vi "PI with FF_0.vi"(0 "Run PI?":bool, 1 "PIcluster":cluster{"SlewRate":dbl, "Kp":dbl, "Ki":dbl}, 2 "FFcluster":cluster{"FF_m":dbl, "FF_b":dbl}, 3 "LimitCluster":T1, 5 "SP":dbl, 7 "Error":dbl, 11 "RevCtrlZero":bool, 13 "Indirect FF":bool) -> (4 "PreSlew":dbl, 8 "Output":dbl)   [LabVIEW 2013]
uses:
  <vilib>/addons/control/pid/pid.llb/PID Output Rate Limiter (DBL).vi
  <vilib>/addons/control/pid/NI_PID_pid.lvlib
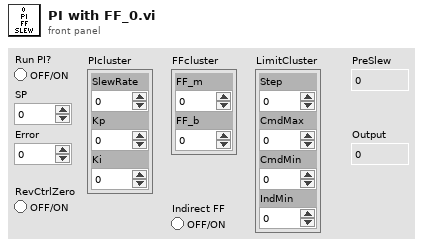
[diagram p1: front panel]
types:
  T1 = cluster{"Step":dbl, "CmdMax":dbl, "CmdMin":dbl, "IndMin":dbl}
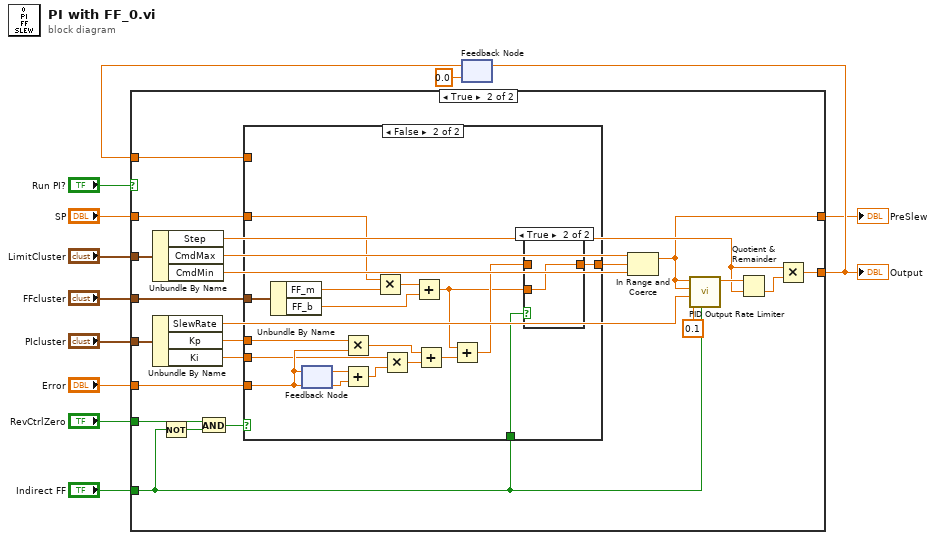
[diagram p0: block diagram]
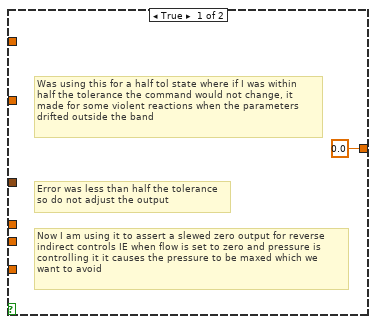
[diagram p3: hidden frame]
diagram:
  n1 = feedback #1(0.0 ("SP")) -> (w4:dbl)
  n2 = case shown="True" "Run PI?" {
    tunnel: [w13 w23] -> w5
    tunnel: "SP" -> [w13 w35]
    tunnel: "Error" -> [_ w34]
    tunnel: "FFcluster" -> [_ w33]
    tunnel: "PIcluster" -> [_ w30]
    tunnel: "LimitCluster" -> [_ w31]
    tunnel: "RevCtrlZero" -> [_ w18]
    tunnel: w4 -> [_ w32]
    tunnel: [w13 w15] -> w2
    tunnel: "Indirect FF" -> [_ w14]
    frame False {
    }
    frame True {
      n3 = Unbundle By Name(w31) -> ("Step"=w24:dbl, "CmdMax"=w21:dbl, "CmdMin"=w20:dbl)
      n4 = Unbundle By Name(w30) -> ("SlewRate"=w25:dbl, "Kp"=w29:dbl, "Ki"=w28:dbl)
      n5 = Not(x=w14) -> (.not. x?=w17:bool)
      n6 = And(x=w18, y=w17) -> (x .and. y?=w16:bool)
      n7 = case shown="False" w16 {
        tunnel: w35 -> [_ w51]
        tunnel: w34 -> [_ w49]
        tunnel: w33 -> [_ w45]
        tunnel: w32 -> [_ _]
        tunnel: w29 -> [_ w42]
        tunnel: w28 -> [_ w41]
        tunnel: [0.0 ("CmdMax") w38] -> w22
        tunnel: w14 -> [_ w40]
        frame True {
          # "Now I am using it to assert a slewed zero output for reverse\nindirect controls IE when flow is set to zero and pressure is\ncontrolling it it causes the pressure to be maxed which we\nwant to avoid"
          # "Was using this for a half tol state where if I was within\nhalf the tolerance the command would not change, it\nmade for some violent reactions when the parameters\ndrifted outside the band"
          # "Error was less than half the tolerance\nso do not adjust the output"
        }
        frame False {
          n8 = Unbundle By Name(w45) -> ("FF_m"=w44:dbl, "FF_b"=w43:dbl)
          n9 = feedback #2(w49) -> (w50:dbl)
          n10 = feedback-in #2(w49) -> ()
          n11 = Multiply(x=w42, y=w49) -> (x*y=w47:dbl)
          n12 = Add(x=w50, y=w49) -> (x+y=w46:dbl)
          n13 = Multiply(x=w51, y=w44) -> (x*y=w53:dbl)
          n14 = Multiply(x=w41, y=w46) -> (x*y=w48:dbl)
          n15 = Add(x=w53, y=w43) -> (x+y=w37:dbl)
          n16 = Add(x=w47, y=w48) -> (x+y=w52:dbl)
          n17 = Add(x=w37, y=w52) -> (x+y=w39:dbl)
          n18 = case shown="True" w40 {
            tunnel: w39 -> [w54 _]
            tunnel: [w54 w55] -> w38
            tunnel: w37 -> [_ w55]
            frame False {
            }
            frame True {
            }
          }
        }
      }
      n19 = In Range and Coerce(upper limit=w21, x=w22, lower limit=w20) -> (coerced(x)=w15:dbl)  [unwired: 1 out]
      n20 = call-poly <vilib>:"PID Output Rate Limiter.vi"("reinitialize? (F)"=w14, "dt (s)"=0.1, "output rate (EGU/min)"=w25, "initial output"=w15, "input (controller output)"=w15) -> ("output"=w27:dbl)  [unwired: 3 in, 1 out]
      n21 = Quotient & Remainder(x=w27, y=w24) -> (floor(x/y)=w26:dbl)  [unwired: 1 out]
      n22 = Multiply(x=w24, y=w26) -> (x*y=w23:dbl)
    }
  }
  "Output" <- w5
  "PreSlew" <- w2
  n23 = feedback-in #1(w5) -> ()
